vi "Front Panel.vi"() -> ()   [LabVIEW 2012]
uses:
  Globalna_Variabla.vi
panel:
  in  "?":enum32{"Prijem", "Ref Num"}(tab)
  out "Sekvenca RS232":dbl[](array[numeric])
  out "Cluster Sekvenca":dbl[](array[numeric])
  out "x = y?":bool
  out "Donja Sekvenca":i32
  in  "Play":dbl
  out "reference out":refnum<vi>
  in  "Device":u32
  in  "stop":bool=TRUE
  out "Boolean 2":bool=TRUE
  out "Podaci sa senzora":T1(graph)
  out "SCORE":dbl
  # "Dodati SW treshold za senzore"
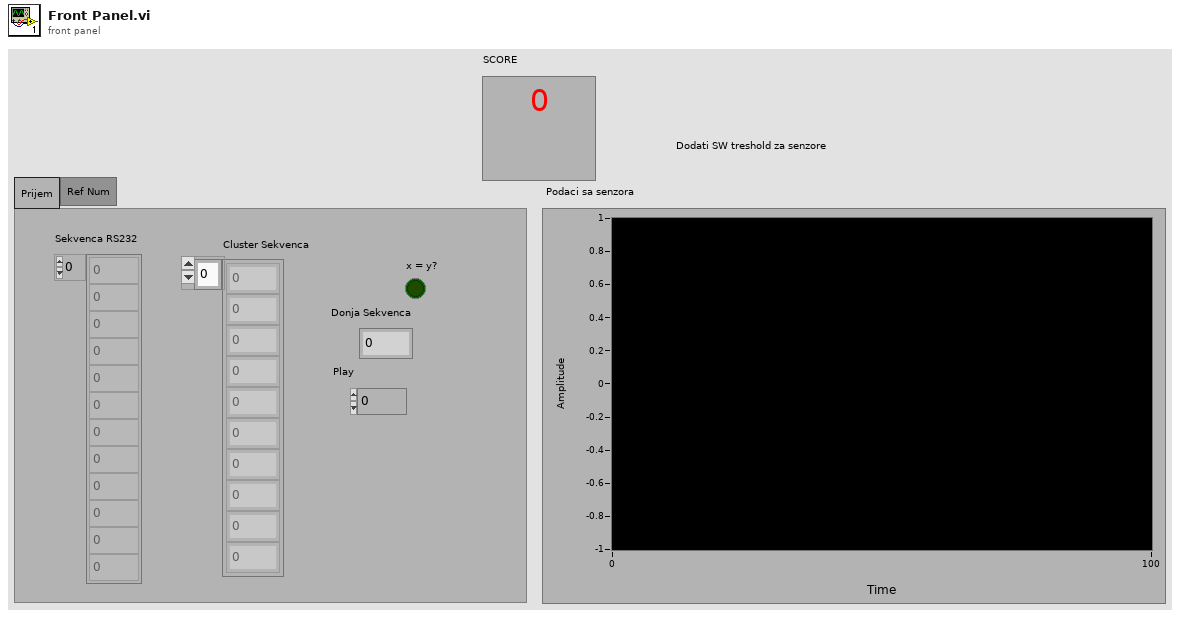
[diagram p1: front panel]
types:
  T1 = cluster{"Numeric":dbl, "Numeric":dbl, "Numeric":dbl, "Numeric":dbl}
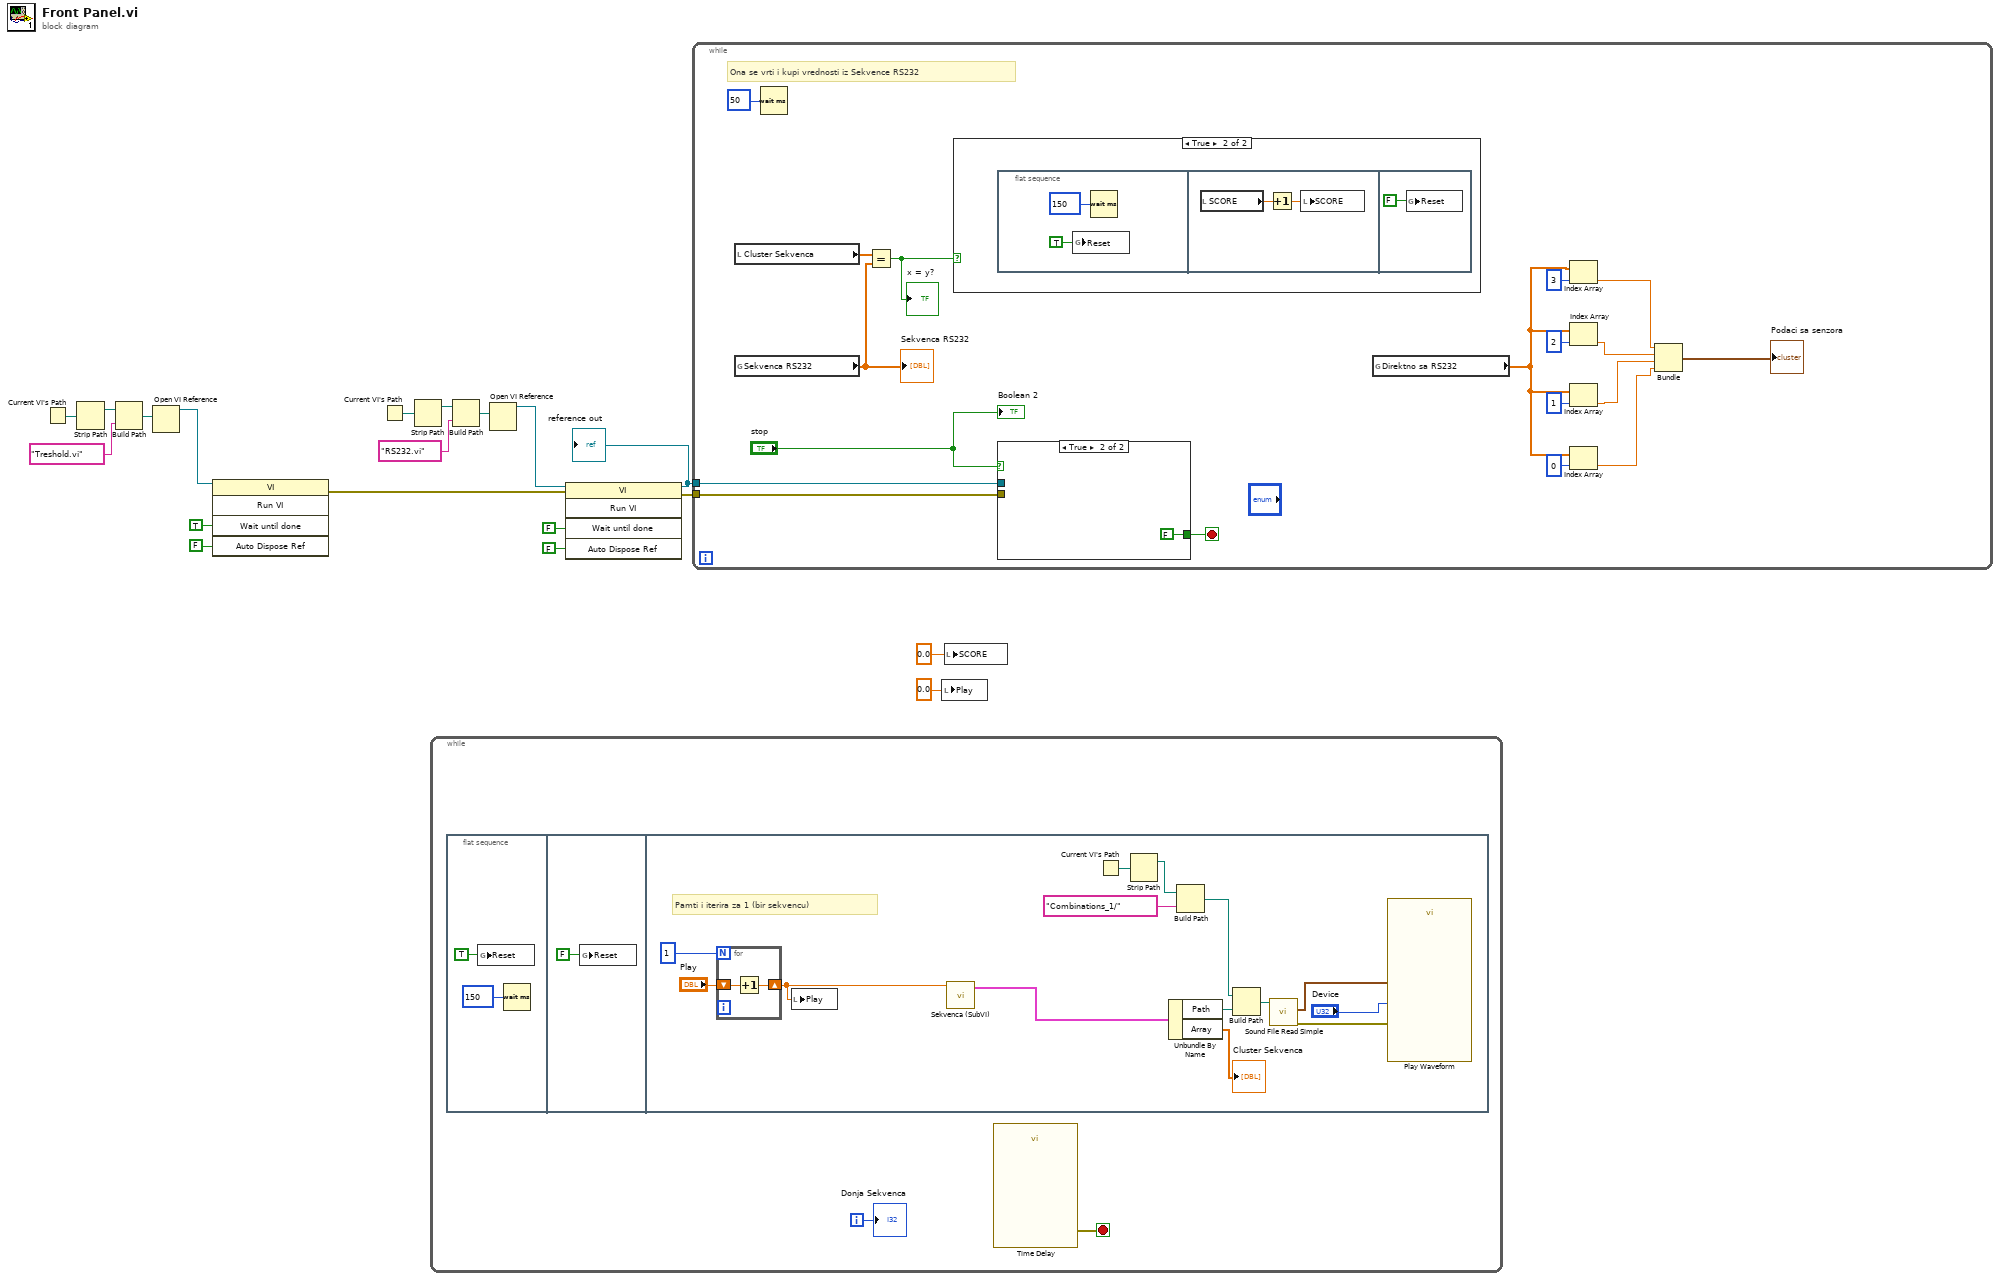
[diagram p0: block diagram]
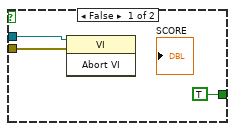
[diagram p3: hidden frame]
diagram:
  n1 = Current VI's Path() -> (path=w4:path)
  n2 = Strip Path(path=w4) -> (stripped path=w3:path)  [unwired: 1 out]
  n3 = Build Path(base path=w3, name or relative path="Treshold.vi") -> (appended path=w2:path)
  n4 = Open VI Reference(vi path=w2) -> (vi reference=w8:refnum<vi>)  [unwired: 5 in, 1 out]
  n5 = invoke class="VI" method="Run VI"(reference=w8, "Wait until done"=TRUE ("Wait Until Done"), "Auto Dispose Ref"=FALSE ("Auto Dispose Reference")) -> (error out=w1:errorcluster)  [unwired: 2 in, 4 out]
  n6 = Current VI's Path() -> (path=w13:path)
  n7 = Strip Path(path=w13) -> (stripped path=w12:path)  [unwired: 1 out]
  n8 = while {
    i -> [w21]
    stop <- w20 stop-if-true
    n9 = flat-sequence {
      frame #0 {
        n10 = global write "Globalna_Variabla.vi" "Reset"(TRUE ("Reset")) -> ()
        n11 = Wait (ms)(milliseconds to wait=u32 150) -> ()  [unwired: 1 out]
      }
      frame #1 {
        n12 = global write "Globalna_Variabla.vi" "Reset"(FALSE ("Reset")) -> ()
      }
      frame #2 {
        # "Pamti i iterira za 1 (bir sekvencu)"
        n13 = for {
          N: 1 -> [_]
          shift-right: [w39] -> w26
          shift-left: "Play" -> [w40]
          n14 = Increment(x=w40) -> (x+1=w39:dbl)
        }
        n15 = local write "Play"(w26) -> ()
        n16 = call "Sekvenca (SubVI).vi"("Ulaz"=w26) -> ("Cluster 41"=w25:cluster{"Path":path, "Array":dbl[]})  [unwired: 10 in]
        n17 = Current VI's Path() -> (path=w33:path)
        n18 = Strip Path(path=w33) -> (stripped path=w34:path)  [unwired: 1 out]
        n19 = Unbundle By Name(w25) -> ("Path"=w35:path, "Array"=→"Cluster Sekvenca":dbl[])
        n20 = Build Path(base path=w34, name or relative path="Combinations_1/") -> (appended path=w36:path)
        n21 = Build Path(base path=w36, name or relative path=w35) -> (appended path=w37:path)
        n22 = call <vilib>:"Sound File Read Simple.vi"("path"=w37) -> ("error out"=w30:errorcluster, "data"=w29:waveform(dbl)[])  [unwired: 7 in, 2 out]
        n23 = call "Play Waveform"("Device"="Device", "Data"=w29, "error in"=w30) -> ()  [unwired: 16 in, 1 out]
      }
    }
    n24 = call "Time Delay"() -> ("error out"=w20:errorcluster)  [unwired: 11 in]
    "Donja Sekvenca" <- w21
  }
  n25 = Build Path(base path=w12, name or relative path="RS232.vi") -> (appended path=w11:path)
  n26 = Open VI Reference(vi path=w11) -> (vi reference=w19:refnum<vi>)  [unwired: 5 in, 1 out]
  n27 = invoke class="VI" method="Run VI"(reference=w19, error in=w1, "Wait until done"=FALSE ("Wait Until Done"), "Auto Dispose Ref"=FALSE ("Auto Dispose Reference")) -> (reference out=w16:refnum<vi>, error out=w15:errorcluster)  [unwired: 1 in, 3 out]
  "reference out" <- w16
  n28 = while {
    tunnel: w16 -> [w56]
    tunnel: w15 -> [w55]
    stop <- w57 stop-if-true
    # "Ona se vrti i kupi vrednosti iz Sekvence RS232"
    n29 = local read "Cluster Sekvenca"() -> (w53:dbl[])
    n30 = global read "Globalna_Variabla.vi" "Sekvenca RS232"() -> (w51:dbl[])
    "Sekvenca RS232" <- w51
    n31 = Wait (ms)(milliseconds to wait=u32 50) -> ()  [unwired: 1 out]
    n32 = Equal?(x=w53, y=w51) -> (x = y?=w52:bool)
    "x = y?" <- w52
    n33 = case shown="True" w52 {
      frame False {
      }
      frame True {
        n34 = flat-sequence {
          frame #0 {
            n35 = global write "Globalna_Variabla.vi" "Reset"(TRUE ("Reset")) -> ()
            n36 = Wait (ms)(milliseconds to wait=u32 150) -> ()  [unwired: 1 out]
          }
          frame #1 {
            n37 = local read "SCORE"() -> (w62:dbl)
            n38 = Increment(x=w62) -> (x+1=w61:dbl)
            n39 = local write "SCORE"(w61) -> ()
          }
          frame #2 {
            n40 = global write "Globalna_Variabla.vi" "Reset"(FALSE ("Reset")) -> ()
          }
        }
      }
    }
    n41 = case shown="True" "stop" {
      tunnel: [TRUE FALSE] -> w57
      tunnel: w56 -> [w65 _]
      tunnel: w55 -> [w64 _]
      frame False {
        n42 = invoke class="VI" method="Abort VI"(reference=w65, error in=w64) -> ()  [unwired: 1 in, 3 out]
      }
      frame True {
      }
    }
    n43 = global read "Globalna_Variabla.vi" "Direktno sa RS232"() -> (w50:dbl[])
    n44 = Index Array(array=w50, index=3) -> (element=w45:dbl)
    n45 = Index Array(array=w50, index=2) -> (element=w44:dbl)
    n46 = Index Array(array=w50, index=1) -> (element=w43:dbl)
    n47 = Index Array(array=w50, index=0) -> (element=w42:dbl)
    n48 = Bundle("Numeric"=w45, "Numeric"=w44, "Numeric"=w43, "Numeric"=w42) -> (→"Podaci sa senzora":T1)  [unwired: 1 in]
    "Boolean 2" <- "stop"
  }
  n49 = local write "Play"(0.0 ("Play")) -> ()
  n50 = local write "SCORE"(0.0 ("SCORE")) -> ()
